vi "Descriptor_GetInfo.vi"(9 "Descriptor":T1) -> (1 "Type":u8 format="%.0x", 2 "name":string)   [LabVIEW 2013, in "OpenDescriptor.lvlib"]
uses:
  OpenDescriptor.lvlib
  OpenDescriptor -- cluster.ctl
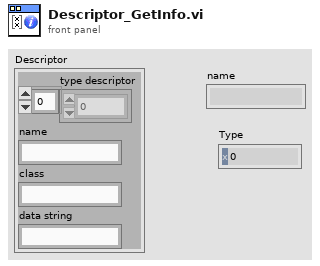
[diagram p1: front panel]
types:
  T1 = typedef "OpenDescriptor.lvlib/OpenDescriptor -- cluster.ctl" = cluster{"type descriptor":i16[], "name":string, "class":string, "data string":string}
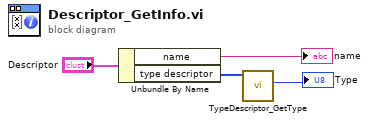
[diagram p0: block diagram]
diagram:
  n1 = Unbundle By Name("Descriptor") -> ("name"=→"name":string, "type descriptor"=w4:i16[])
  n2 = call "TypeDescriptor_GetType.vi"("type descriptor"=w4) -> ("Type"=→"Type":u8)  [unwired: 9 in, 1 out]
